vi "Move to IR.vi"(0 "SS Index (3)":i32=3, 4 "Timeout (ms)":u32=3000, 5 "Drive 2":T3, 6 "Signal Strength":u8=115, 7 "Drive 1":T3, 8 "Direction":i16=7, 9 "Power/Speed 2":i8, 10 "Power/Speed 1":i8, 11 "NXT In":T1) -> (1 "Data Logging":cluster{i32, i32, "32bit integer":i32}[](array[cluster]), 3 "NXT Out":T1)   [LabVIEW 2010, in "4150_RingItUp_State.lvrbt"]
uses:
  4150_RingItUp_State/4150_RingItUp_State.lvrbt
  <vilib>/NXT/Subs/MotorXNode.DC Motor Type.ctl
  <vilib>/NXT/Subs/LVHSConnector.ctl
  <vilib>/NXT/HiTechnic/HiTechnic Controls/HiTechnic Port.ctl
  <vilib>/NXT/Block Support/NXT_InputPort.ctl
  <vilib>/NXT/NXTIO Xnodes/NXTIOXNode/NXTIO.xnode
  <vilib>/NXT/Subs/MotorXNode.2DCMotor.ctl
  <vilib>/NXT/NXTIO Xnodes/NXTIONodeSubVIs/TETRIX IO Move DC Motors.vi
  <vilib>/NXT/NXTIO Xnodes/NXTIONodeSubVIs/TETRIX IO Stop DC Motors.vi
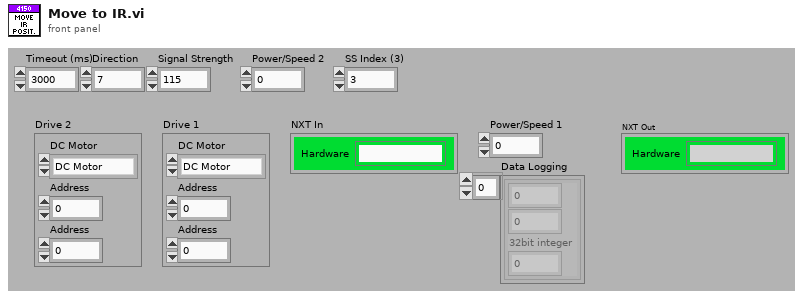
[diagram p1: front panel]
types:
  T1 = typedef "LVHSConnector.ctl" = cluster{"Hardware":string, "Flattened String":string}
  T2 = typedef "MotorXNode.DC Motor Type.ctl" = enum16{"DC Motor"}
  T3 = cluster{"DC Motor":T2, "Address":i16, "Address":i16}
  T4 = typedef "HiTechnic Port.ctl" = cluster{"Port":T5, "MUX Port":u8}
  T5 = typedef "NXT_InputPort.ctl" = u8
  T6 = cluster{"Direction (0-9)":i16, "Signal Strength (Array)":u8[]}
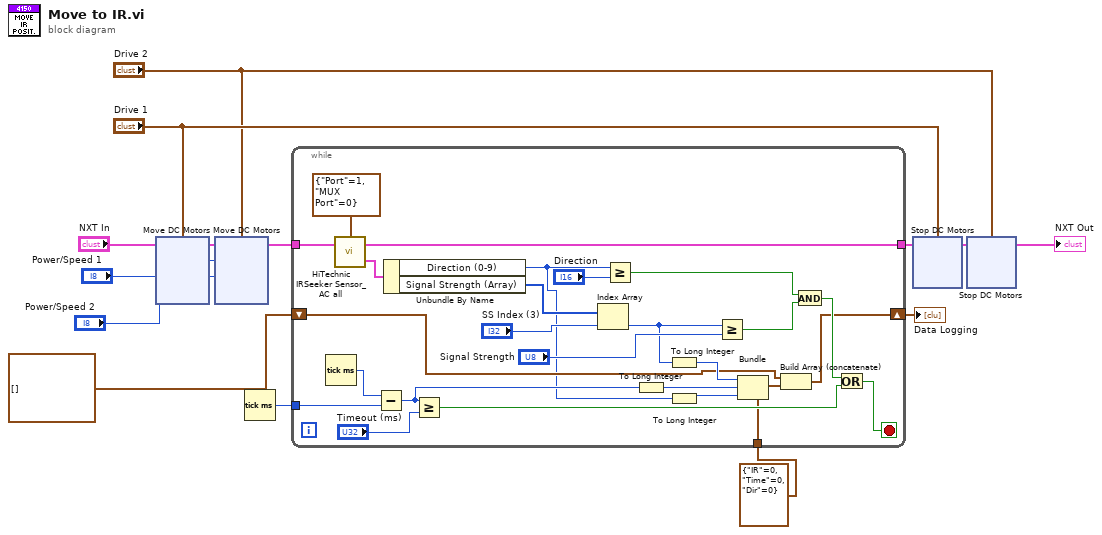
[diagram p0: block diagram]
diagram:
  n1 = xnode "Move DC Motors"("Power/Speed 2"="Power/Speed 2", "Power/Speed 1"="Power/Speed 1", "Motors"="Drive 1", "NXT"="NXT In") -> ("NXT"=w8:T1)
  n2 = xnode "Move DC Motors"("Power/Speed 2"="Power/Speed 2", "Power/Speed 1"="Power/Speed 1", "Motors"="Drive 2", "NXT"=w8) -> ("NXT"=w10:T1)
  n3 = Tick Count (ms)() -> (millisecond timer value=w11:u32)
  n4 = while {
    tunnel: w10 -> [w40]
    tunnel: w11 -> [w31]
    tunnel: [w27] -> w12
    shift-right: [w24] -> w2
    shift-left: cluster{"IR":i32, "Time":i32, "Dir":i32}[] [] -> [w18]
    tunnel: cluster{"IR":i32, "Time":i32, "Dir":i32} {"IR"=0, "Time"=0, "Dir"=0} -> [w15]
    stop <- w26 stop-if-true
    n5 = Tick Count (ms)() -> (millisecond timer value=w32:u32)
    n6 = call <vilib>:"HiTechnic IRSeeker Sensor_AC all.vi"("NXT"=w40, "Port/MUX"=T4 {"Port"=1, "MUX Port"=0}) -> ("All Info"=w39:T6, "NXT"=w27:T1)  [unwired: 1 in]
    n7 = Subtract(x=w32, y=w31) -> (x-y=w22:u32)
    n8 = Unbundle By Name(w39) -> ("Direction (0-9)"=w16:i16, "Signal Strength (Array)"=w37:u8[])
    n9 = Greater Or Equal?(x=w22, y="Timeout (ms)") -> (x >= y?=w28:bool)
    n10 = Index Array(array=w37, index="SS Index (3)") -> (element=w23:u8)
    n11 = Greater Or Equal?(x=w16, y="Direction") -> (x >= y?=w34:bool)
    n12 = To Long Integer(number=w22) -> (32bit integer=w21:i32)
    n13 = To Long Integer(number=w23) -> (32bit integer=w20:i32)
    n14 = To Long Integer(number=w16) -> (32bit integer=w17:i32)
    n15 = Greater Or Equal?(x=w23, y="Signal Strength") -> (x >= y?=w33:bool)
    n16 = Bundle(cluster=w15, "IR"=w20, "Time"=w21, "Dir"=w17) -> (w19:cluster{"IR":i32, "Time":i32, "Dir":i32})
    n17 = Build Array (concatenate)(w18, w19) -> (w24:cluster{"IR":i32, "Time":i32, "Dir":i32}[])
    n18 = And(x=w34, y=w33) -> (x .and. y?=w29:bool)
    n19 = Or(x=w29, y=w28) -> (x .or. y?=w26:bool)
  }
  "Data Logging" <- w2
  n20 = xnode "Stop DC Motors"("Motors"="Drive 1", "NXT"=w12) -> ("NXT"=w13:T1)
  n21 = xnode "Stop DC Motors"("Motors"="Drive 2", "NXT"=w13) -> ("NXT"=→"NXT Out":T1)
